vi "BeltDriveAutoControl.vi"(5 "Button 10":bool, 7 "Button 11":bool, 8 "botMotor":i8, 10 "topMotor":i8, 11 "BeltDriveAutoOnOff":bool) -> (1 "botMotor":dbl, 3 "topMotor":dbl)   [LabVIEW 2012]
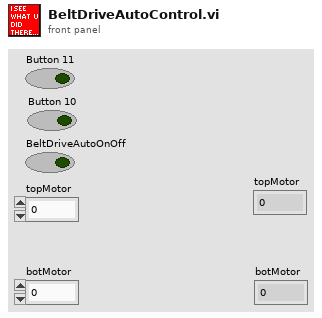
[diagram p1: front panel]
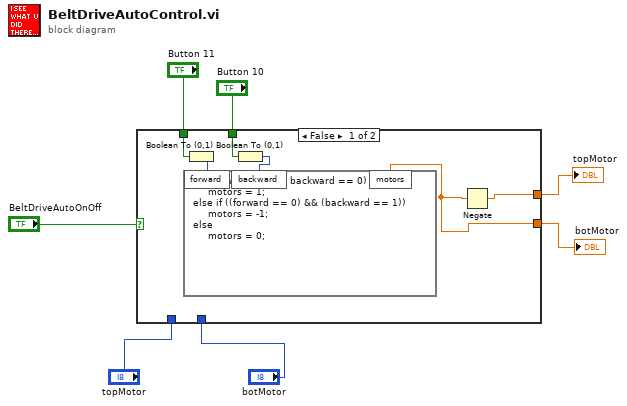
[diagram p0: block diagram]
diagram:
  n1 = case shown="False" "BeltDriveAutoOnOff" {
    tunnel: "topMotor" -> [_ w15]
    tunnel: "botMotor" -> [_ w14]
    tunnel: [w9 w15] -> w2
    tunnel: [w8 w14] -> w1
    tunnel: "Button 11" -> [w11 _]
    tunnel: "Button 10" -> [w10 _]
    frame False {
      n2 = Boolean To (0,1)(Boolean=w11) -> (0, 1=w13:i16)
      n3 = Boolean To (0,1)(Boolean=w10) -> (0, 1=w12:i16)
      n4 = formula code="if (forward == 1 && backward == 0)\n     motors = 1;\nelse if ((forward == 0) && (backward == 1))\n     motors = -1;\nelse\n     motors = 0;"("forward"=w13, "backward"=w12) -> ("motors"=w8:dbl)
      n5 = Negate(x=w8) -> (-x=w9:dbl)
    }
    frame True {
    }
  }
  "topMotor" <- w2
  "botMotor" <- w1
